vi "BUILD_uninstall core.vi"(10 "LabVIEW Version":string, 11 "appended path":path) -> (0 "error out":errorcluster)   [LabVIEW 2013]
uses:
  <vilib>/JKI/VIPM API/VIPM API_vipm_api.lvlib
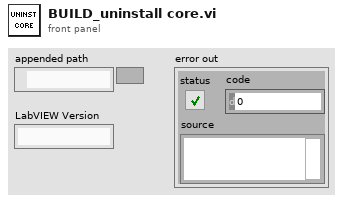
[diagram p1: front panel]
types:
  T1 = typedef "VIPM API_vipm_api.lvlib/Library Contents Cluster_vipm_api.ctl" = cluster{"Package Name":string, "Version":string, "Display Name":string, "Repository Name":string, "Company Name":string, "License Type":string, "Installed":bool, "Deprecated":bool, "Dependency or Conflict Problem":bool, "Downloaded":bool}
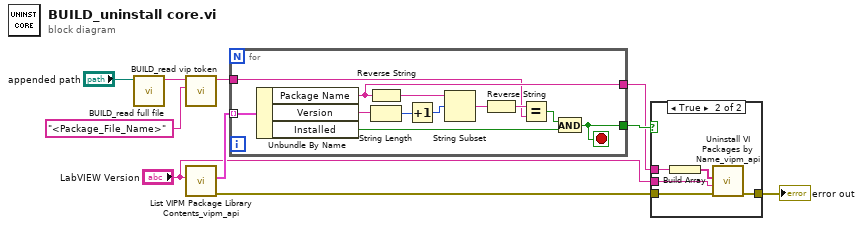
[diagram p0: block diagram]
diagram:
  n1 = call "BUILD_read full file.vi"("vip file"="appended path") -> ("data"=w9:string)  [unwired: 9 in, 1 out]
  n2 = call "BUILD_read vip token.vi"("regular expression"="<Package_File_Name>", "data"=w9) -> ("trimmed string"=w8:string)  [unwired: 9 in]
  n3 = call <vilib>:"List VIPM Package Library Contents_vipm_api.vi"("LabVIEW Version"="LabVIEW Version") -> ("error out"=w4:errorcluster, "Library Contents []"=w3:T1[])  [unwired: 9 in]
  n4 = for {
    tunnel: w3 -> [w22] mode=indexing
    tunnel: [w16] -> w5
    tunnel: [w12] -> w6
    tunnel: w8 -> [w11]
    stop <- w12 stop-if-true
    n5 = Unbundle By Name(w22) -> ("Package Name"=w16:string, "Version"=w21:string, "Installed"=w13:bool)
    n6 = Reverse String(1:w16) -> (0:w18:string)
    n7 = String Length(string=w21) -> (length=w20:i32)
    n8 = Increment(x=w20) -> (x+1=w19:i32)
    n9 = String Subset(string=w18, offset (0)=w19) -> (substring=w17:string)  [unwired: 1 in]
    n10 = Reverse String(1:w17) -> (0:w15:string)
    n11 = Equal?(x=w15, y=w11) -> (x = y?=w14:bool)
    n12 = And(x=w14, y=w13) -> (x .and. y?=w12:bool)
  }
  n13 = case shown="True" w6 {
    tunnel: [w23 w27] -> w1
    tunnel: "LabVIEW Version" -> [_ w26]
    tunnel: w4 -> [w23 w25]
    tunnel: w5 -> [_ w24]
    frame False {
    }
    frame True {
      n14 = Build Array(w24) -> (w28:string[])
      n15 = call <vilib>:"Uninstall VI Packages by Name_vipm_api.vi"("error in (no error)"=w25, "LabVIEW Version"=w26, "Package Names to Uninstall []"=w28) -> ("error out"=w27:errorcluster)  [unwired: 8 in]
    }
  }
  "error out" <- w1
